vi "HMS_Firmware_Manager_II_Convert.vi"(5 "error in (no error)":errorcluster) -> (12 "Network Updated":bool, 13 "Pass":bool, 14 "standard error":string, 15 "standard output":string, 16 "Network Changed":bool, 17 "Module Detected":bool, 18 "Latest Firmware Found":bool, 19 "error out":errorcluster)   [LabVIEW 2016]
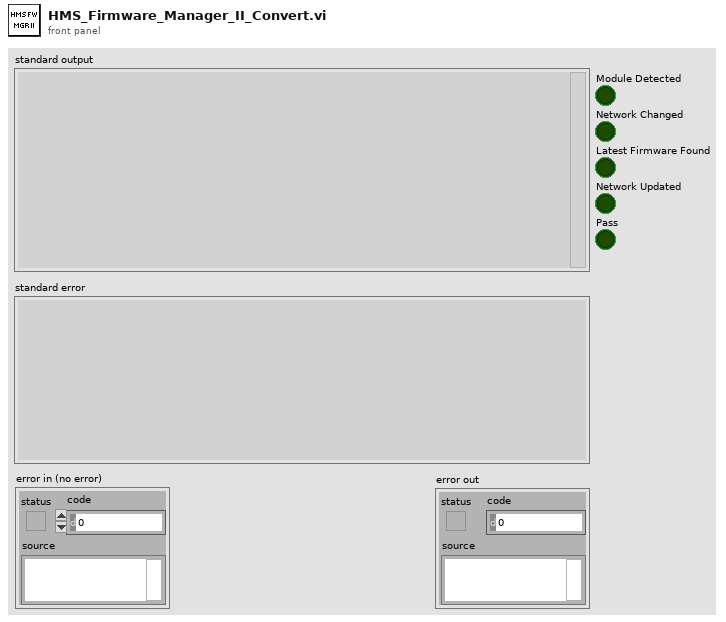
[diagram p1: front panel]
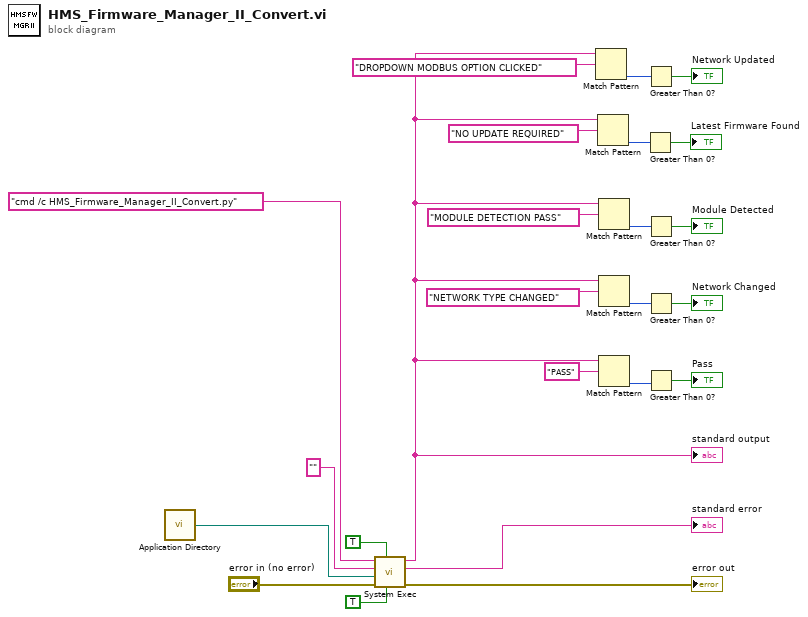
[diagram p0: block diagram]
diagram:
  n1 = call <vilib>:"Application Directory.vi"() -> ("Application Directory"=w5:path)
  n2 = call <vilib>:"System Exec.vi"("run minimized? (F)"=TRUE, "wait until completion? (T)"=TRUE ("run minimized? (F)"), "error in (no error)"="error in (no error)", "working directory"=w5, "standard input"="", "command line"="cmd /c HMS_Firmware_Manager_II_Convert.py" ("name or relative path")) -> ("error out"=→"error out":errorcluster, "standard error"=→"standard error":string, "standard output"=w3:string)  [unwired: 2 in, 1 out]
  "standard output" <- w3
  n3 = Match Pattern(string=w3, regular expression="DROPDOWN MODBUS OPTION CLICKED") -> (offset past match=w1:i32)  [unwired: 1 in, 3 out]
  n4 = Match Pattern(string=w3, regular expression="NO UPDATE REQUIRED") -> (offset past match=w8:i32)  [unwired: 1 in, 3 out]
  n5 = Match Pattern(string=w3, regular expression="MODULE DETECTION PASS") -> (offset past match=w11:i32)  [unwired: 1 in, 3 out]
  n6 = Match Pattern(string=w3, regular expression="NETWORK TYPE CHANGED") -> (offset past match=w12:i32)  [unwired: 1 in, 3 out]
  n7 = Match Pattern(string=w3, regular expression="PASS") -> (offset past match=w17:i32)  [unwired: 1 in, 3 out]
  n8 = Greater Than 0?(x=w8) -> (x > 0?=→"Latest Firmware Found":bool)
  n9 = Greater Than 0?(x=w1) -> (x > 0?=→"Network Updated":bool)
  n10 = Greater Than 0?(x=w11) -> (x > 0?=→"Module Detected":bool)
  n11 = Greater Than 0?(x=w12) -> (x > 0?=→"Network Changed":bool)
  n12 = Greater Than 0?(x=w17) -> (x > 0?=→"Pass":bool)
